vi "DIO initialize.vi"(8 "error in":errorcluster, 11 "FPGA VI Reference In":refnum<k20>) -> (0 "error out":errorcluster, 3 "FPGA VI Reference Out":refnum<k20>)   [LabVIEW 2017]
uses:
  <vilib>/rvi/interface/common/niFpgaWaitOnOcc.vi
  <vilib>/Utility/error.llb/Error Cluster From Error Code.vi
  <vilib>/FPGAPlugInAG/Dynamic/niLvFpga_Run_Dynamic.vi
  <vilib>/rvi/interface/nirviMethod/nirviMethod.xnode
  <vilib>/FPGAPlugInAG/Dynamic/niLvFpga_ConfigureFifo_Dynamic.vi
  <vilib>/rvi/errors/niLvFpgaMergeErrorWithErrorCode.vi
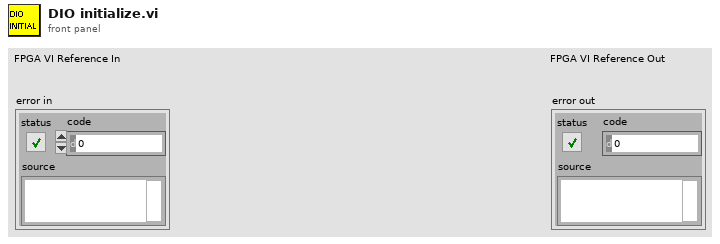
[diagram p1: front panel]
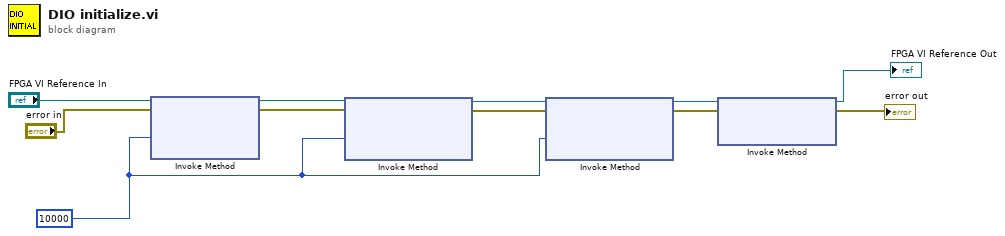
[diagram p0: block diagram]
diagram:
  w5 = u32 10000 ("Requested Depth")
  n1 = xnode "Invoke Method"("FPGA VI Reference In"="FPGA VI Reference In", "error in"="error in", "Requested Depth"=w5) -> ("FPGA VI Reference Out"=w9:refnum<k20>, "error out"=w8:errorcluster)  [unwired: 1 out]
  n2 = xnode "Invoke Method"("FPGA VI Reference In"=w9, "error in"=w8, "Requested Depth"=w5) -> ("FPGA VI Reference Out"=w7:refnum<k20>, "error out"=w6:errorcluster)  [unwired: 1 out]
  n3 = xnode "Invoke Method"("FPGA VI Reference In"=w7, "error in"=w6, "Requested Depth"=w5) -> ("FPGA VI Reference Out"=w4:refnum<k20>, "error out"=w3:errorcluster)  [unwired: 1 out]
  n4 = xnode "Invoke Method"("FPGA VI Reference In"=w4, "error in"=w3) -> ("FPGA VI Reference Out"=→"FPGA VI Reference Out":refnum<k20>, "error out"=→"error out":errorcluster)  [unwired: 1 in]
